vi "Close Document.vi"(8 "error in (no error)":errorcluster, 11 "Document in":refnum<class "npoiDocument.lvclass">) -> (0 "error out":errorcluster)   [LabVIEW 2017, in "NPOI_Document.lvlib" / "npoiDocument.lvclass"]
doc: "Closes the underlying <b>Document in</b> resources, from which the Document was created.\n\nNotes:\n - Once this has been called, no further operations, updates or reads should be performed on the <b>Document</b>."
uses:
  npoiDocument.lvclass
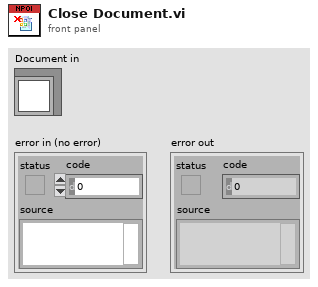
[diagram p1: front panel]
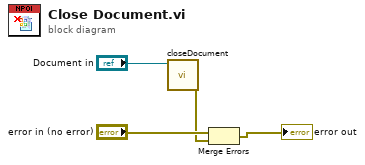
[diagram p0: block diagram]
diagram:
  n1 = call-dynamic "closeDocument.vi"("npoiDocument in"="Document in") -> ("error out"=w1:errorcluster)  [unwired: 9 in, 1 out]
  n2 = Merge Errors("error in (no error)", w1) -> (→"error out":errorcluster)
